vi "Init.vi"(8 "error in (no error)":errorcluster, 10 "PS Driver.lvlib:PS Driver.lvclass":refnum<class "PS Driver.lvclass">, 11 "PS Control Actor in":refnum<class "PS Control Actor.lvclass">) -> (0 "error out":errorcluster, 3 "Actor's Enqueuer":refnum<class "Message Enqueuer.lvclass">)   [LabVIEW 2024, in "PS Control Actor.lvlib" / "PS Control Actor.lvclass"]
uses:
  PS Control Actor.lvclass
  <vilib>/ActorFramework/Message Enqueuer/Message Enqueuer.lvclass
  C:/Program Files/National Instruments/LabVIEW 2024/vi.lib/ActorFramework/Actor/Actor.lvclass
  PS Driver/PS Driver.lvclass
  PS Control Actor.lvclass/PS Control Actor.ctl
  <vilib>/ActorFramework/Message Enqueuer/Message Enqueuer.lvclass/Message Enqueuer.ctl
  PS Control Actor Messages/Start or stop continuous status updates Msg/Start or stop continuous status updates Msg.lvclass/Start or stop continuous status updates Msg.ctl
  <vilib>/ActorFramework/Message Enqueuer/Enqueue.vi
  PS Control Actor Messages/Update Mode Menu Items Msg/Update Mode Menu Items Msg.lvclass
  C:/Program Files/National Instruments/LabVIEW 2024/vi.lib/ActorFramework/Message/Message.lvclass
  PS Control Actor Messages/Start or stop continuous status updates Msg/Start or stop continuous status updates Msg.lvclass
  PS Control Actor Messages/Init from PS Msg/Init from PS Msg.lvclass
  <vilib>/ActorFramework/Message Priority Queue/Priority Enqueue.vi
  <vilib>/ActorFramework/Actor/Actor.lvclass
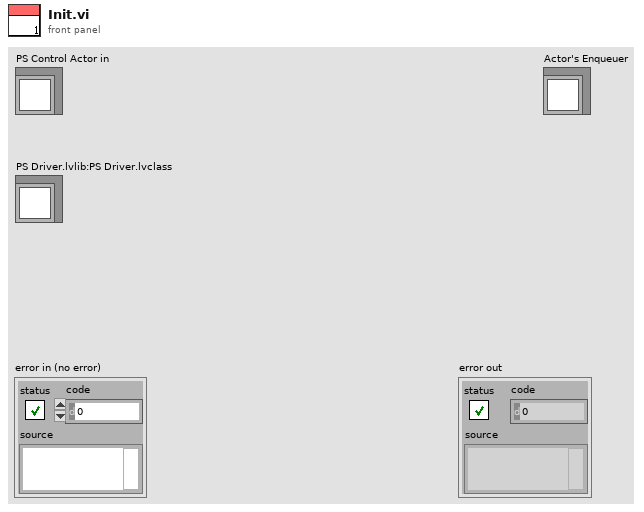
[diagram p1: front panel]
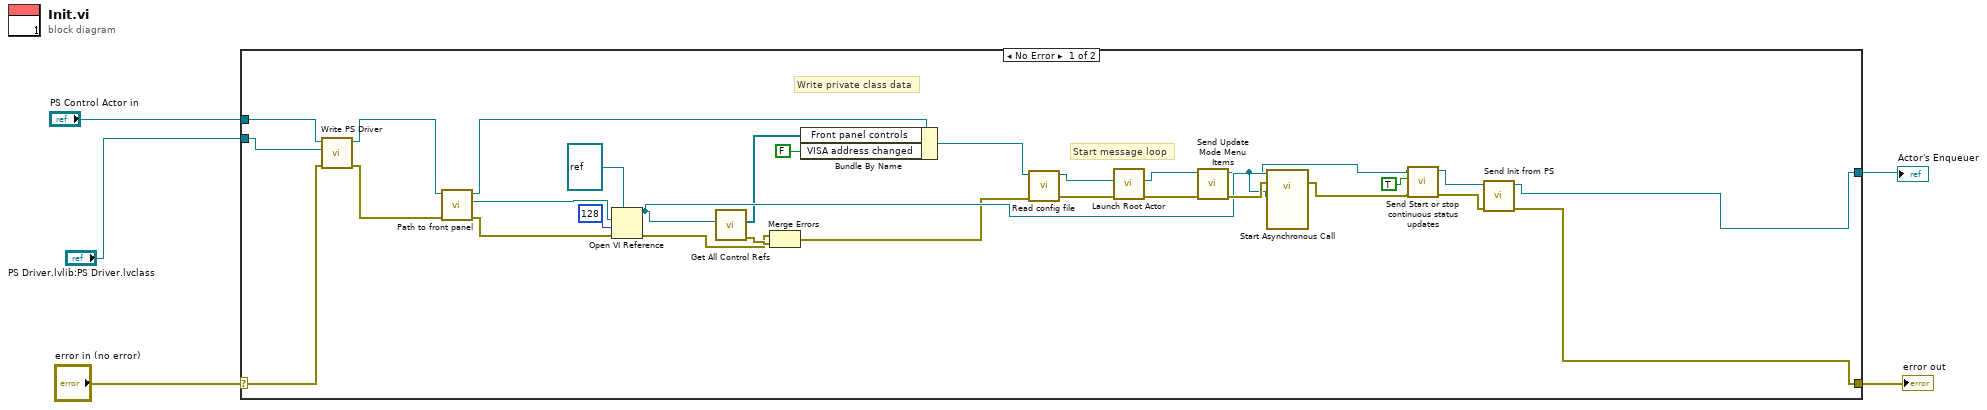
[diagram p0: block diagram]
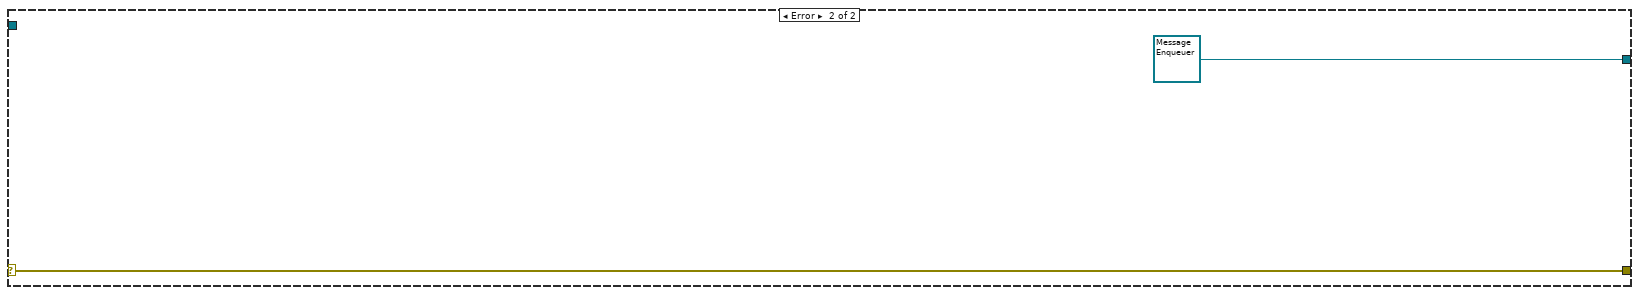
[diagram p2: hidden frame]
diagram:
  n1 = case shown="No Error" "error in (no error)" {
    selector: "error in (no error)" -> [w12 w36]
    tunnel: [w7 w36] -> w5
    tunnel: "PS Control Actor in" -> [w14 _]
    tunnel: [w6 refnum<class "Message Enqueuer.lvclass"> refnum ("Actor's Enqueuer")] -> w3
    tunnel: "PS Driver.lvlib:PS Driver.lvclass" -> [w15 _]
    frame No Error {
      # "Start message loop"
      # "Write private class data"
      n2 = call-dynamic "Write PS Driver.vi"("error in (no error)"=w12, "PS Driver.lvlib:PS Driver.lvclass"=w15, "PS Control Actor in"=w14) -> ("error out"=w11:errorcluster, "PS Control Actor out"=w13:refnum<class "PS Control Actor.lvclass">)  [unwired: 7 in]
      n3 = call-dynamic "Path to front panel.vi"("error in (no error)"=w11, "PS Control Actor in"=w13) -> ("error out"=w27:errorcluster, "Path to front panel VI"=w24:path, "PS Control Actor out"=w10:refnum<class "PS Control Actor.lvclass">)  [unwired: 7 in]
      n4 = Open VI Reference(type specifier VI Refnum (for type only)=refnum<vi> refnum, vi path=w24, options=128, error in (no error)=w27) -> (vi reference=w21:refnum<vi>, error out=w22:errorcluster)  [unwired: 2 in]
      n5 = call "Get All Control Refs.vi"("vi reference"=w21) -> ("All Controls"=w16:refnum<vi>[], "error out"=w26:errorcluster)  [unwired: 5 in, 1 out]
      n6 = Merge Errors(w22, w26) -> (w17:errorcluster)
      n7 = Bundle By Name(cluster=w10, "Front panel controls"=w16, "VISA address changed"=FALSE) -> (w33:refnum<class "PS Control Actor.lvclass">)
      n8 = call "Read config file.vi"("error in (no error)"=w17, "PS Control Actor in"=w33) -> ("error out"=w31:errorcluster, "PS Control Actor out"=w32:refnum<class "PS Control Actor.lvclass">)  [unwired: 8 in]
      n9 = call <vilib>:"Launch Root Actor.vi"("error in (no error)"=w31, "Actor"=w32) -> ("error out"=w29:errorcluster, "Actor's Enqueuer"=w30:refnum<class "Message Enqueuer.lvclass">)  [unwired: 8 in]
      n10 = call "Send Update Mode Menu Items.vi"("error in (no error)"=w29, "Message Enqueuer"=w30) -> ("error out"=w23:errorcluster, "Message Enqueuer out"=w20:refnum<class "Message Enqueuer.lvclass">)  [unwired: 8 in]
      n11 = call-by-ref "Start Asynchronous Call"(reference=w21, error in=w23, "Message Enqueuer"=w20) -> (error out=w18:errorcluster)  [unwired: 11 in, 1 out]
      n12 = call "Send Start or stop continuous status updates.vi"("error in (no error)"=w18, "Continuous status updates"=TRUE, "Message Enqueuer"=w20) -> ("error out"=w8:errorcluster, "Message Enqueuer out"=w9:refnum<class "Message Enqueuer.lvclass">)  [unwired: 7 in]
      n13 = call "Send Init from PS.vi"("error in (no error)"=w8, "Message Enqueuer"=w9) -> ("error out"=w7:errorcluster, "Message Enqueuer out"=w6:refnum<class "Message Enqueuer.lvclass">)  [unwired: 8 in]
    }
    frame Error {
    }
  }
  "error out" <- w5
  "Actor's Enqueuer" <- w3
